vi "Photometer calibration.vi"(11 "Photometer index":i32) -> ()   [LabVIEW 2019]
uses:
  Photometer calibration data.ctl
  toolbar icons/Export pcm.ctl
  toolbar icons/Open calibration.ctl
  toolbar icons/Save calibration.ctl
  DAQ configuration/Sensor buffer command.ctl
  Process Controller 3.0/Calibration and Function folders.ctl
panel:
  in  "Tab Control":enum32{"Analysis", "Help"}(tab)
  out "Absorbance linear fit":cluster{"Best Linear Fit":dbl[], dbl[]}[](graph)
  in  "units":string
  in  "Add Standard":bool
  in  "Clear Standards":bool
  out "Voltage":sgl[unit] format="%.3f"
  out "Concentration":dbl format="%_3f"
  out "XY Graph":cluster{dbl[], dbl[]}[](graph)
  out "A":dbl format="%_3f"
  in  "data averaging (s)":sgl=5.0 format="%.1f"
  in  "Standards":cluster{"Concentration":dbl, "Voltage":dbl}[](array[cluster])=[{"Concentration"=2.0, "Voltage"=2.35551381111145}, {"Concentration"=5.0, "Voltage"=1.50419282913208}, {"Concentration"=10.0, "Voltage"=0.7342819571495056}, {"Concentration"=20.0, "Voltage"=0.23017707467079163}, {"Concentration"=50.0, "Voltage"=0.09496632218360901}] caption="Concentration                        Voltage"
  out "Dark Voltage":dbl=0.09145960211753845
  out "Blank Voltage":dbl=3.127514600753784
  in  "Read\nStandard":bool[](array[boolean])
  in  "Read Dark":bool
  in  "Read Blank":bool
  in  "OK Button":bool
  in  "Cancel":bool
  out "slope":dbl
  out "intercept":dbl
  out "R-square":dbl
  in  "export":T1
  in  "Open calibration":T2
  in  "Save calibration":T3
  out "Photometer data in":T4
  out "Quit":bool
  # "Dark voltage is obtained by turning off the LED light or by completely blocking the sensor. Use an opaque object (not your finger).\nBlank is the same as a standard with zero concentration of the constituent that is being measured.\n\nYou can add or delete standards by right clicking and selecting Insert Element Before or Delete Element."
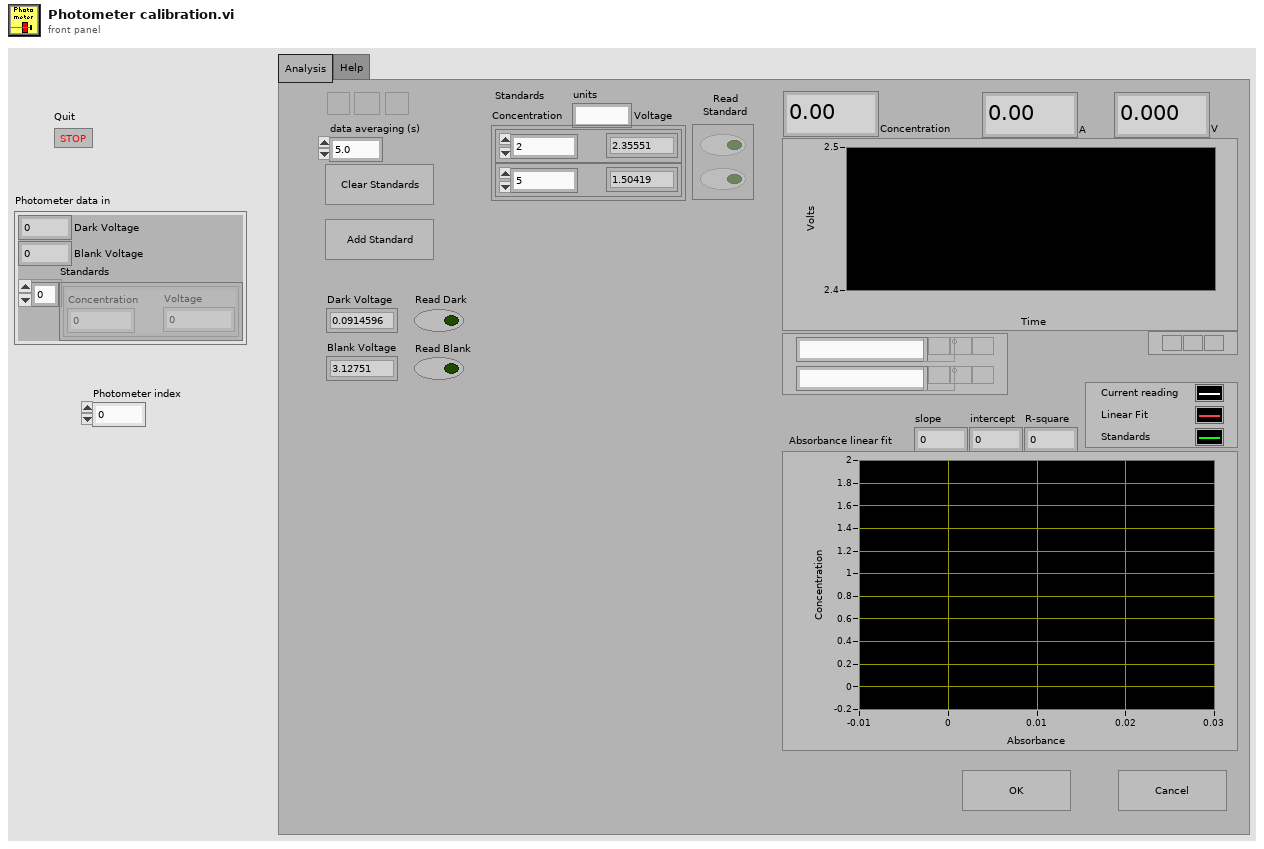
[diagram p1: front panel]
types:
  T1 = typedef "Export pcm.ctl" = bool
  T2 = typedef "Open calibration.ctl" = bool
  T3 = typedef "Save calibration.ctl" = bool
  T4 = typedef "Photometer calibration data.ctl" = cluster{"Dark Voltage":dbl, "Blank Voltage":dbl, "Standards":cluster{"Concentration":dbl, "Voltage":dbl}[]}
  T5 = typedef "Sensor buffer command.ctl" = enum16{"read average", "read recent", "read all", "write", "set buffer size", "Read channel config", "Write channel config", "clear"}
  T6 = typedef "Calibration and Function folders.ctl" = enum16{"Sensors", "Functions", "Config File", "PublicAppFolder", "New ini File", "Set Config File", "Delete ini File"}
  T7 = typedef "Channel config.ctl" = cluster{"Channel Indices":T8[], "AI Max voltage":dbl[], "Calibration matrix":T9}
  T8 = typedef "channel identifier.ctl" = u16
  T9 = typedef "calib array.ctl" = T10[]
  T10 = typedef "conversion.ctl" = cluster{"conversion matrix":sgl[][], "units":string, "name":string, "scale type":T11, "offset (volts)":dbl, "second channel":i8, "correspondence table":T12, "offset (physical units)":dbl, "pH scale":T13, "D.O.":T14, "Photometer data":T4}
  T11 = typedef "scale type.ctl" = enum16{"Volts", "Polynomial", "Correspondence Table", "pH", "Dissolved Oxygen", "Quadratic", "Photometer"}
  T12 = typedef "correspondence table.ctl" = cluster{"physical units":dbl, "volts":dbl}[]
  T13 = typedef "pH scale.ctl" = cluster{"Buffers":cluster{"Buffer":dbl, "Calibrated":bool, "V/T":dbl}[], "Temperature":dbl}
  T14 = typedef "DO scale.ctl" = cluster{"Temperature":dbl, "K":dbl, "barometric pressure":dbl}
  T15 = typedef "Sensor data.ctl" = cluster{" Sensor array":T16[], "Time":dbl}
  T16 = typedef "sensor cluster.ctl" = cluster{"voltage":sgl, "scaled":sgl, "units":string, "Out of Range":bool}
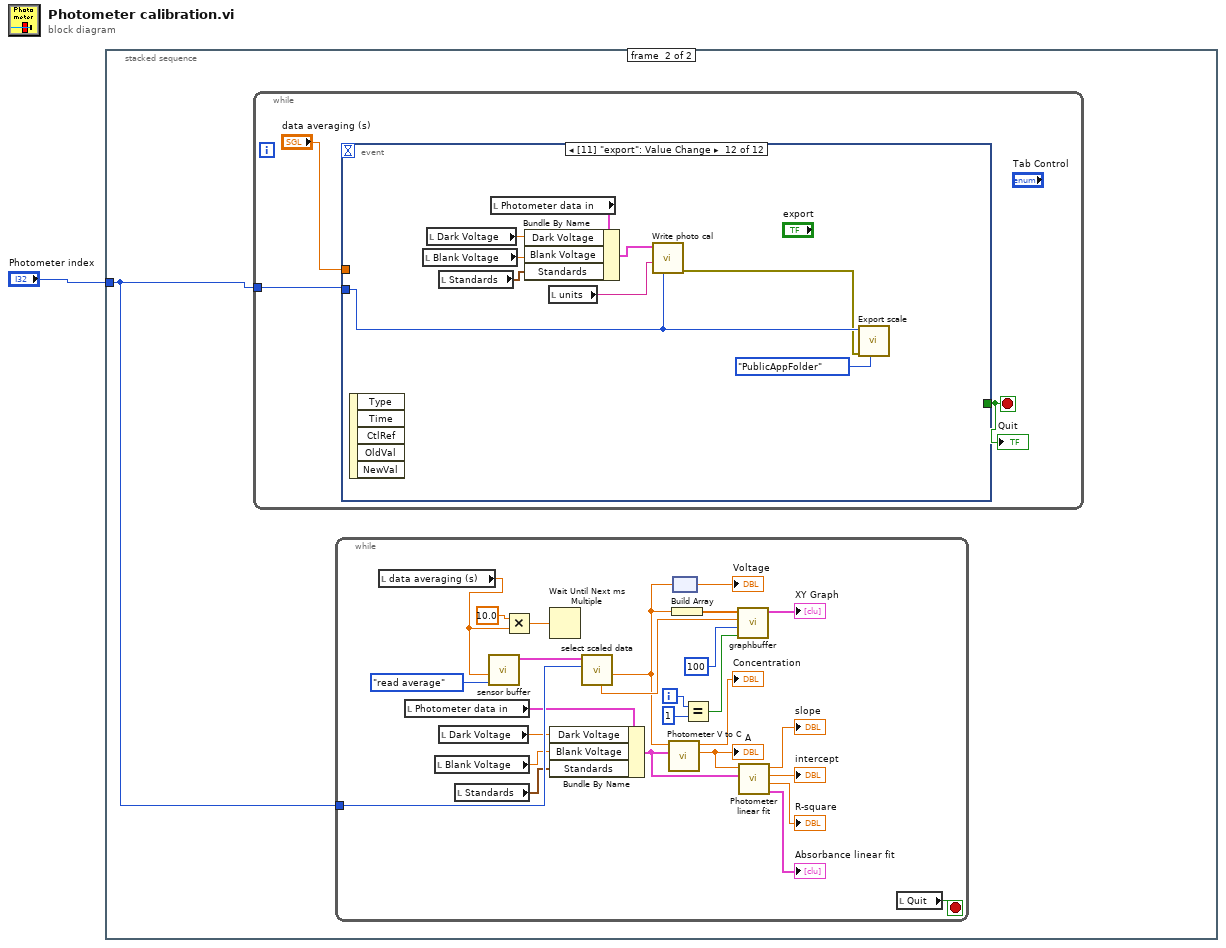
[diagram p0: block diagram]
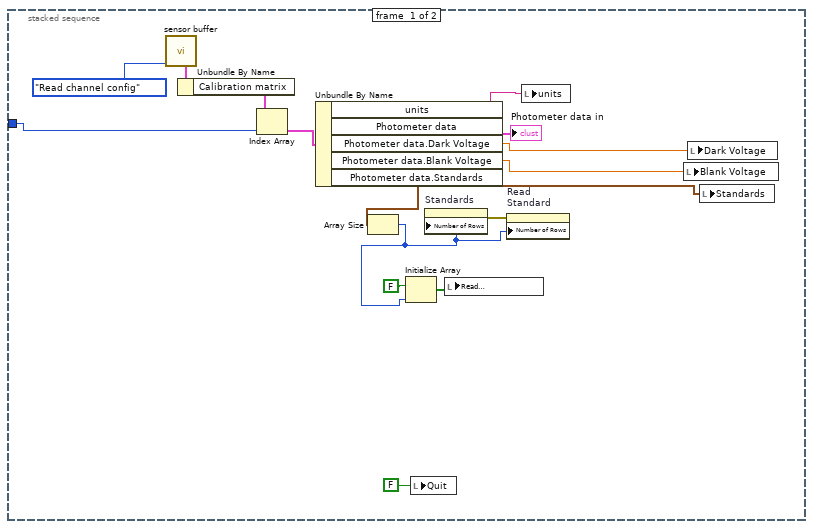
[diagram p2: hidden frame]
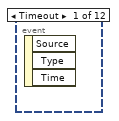
[diagram p3: hidden frame]
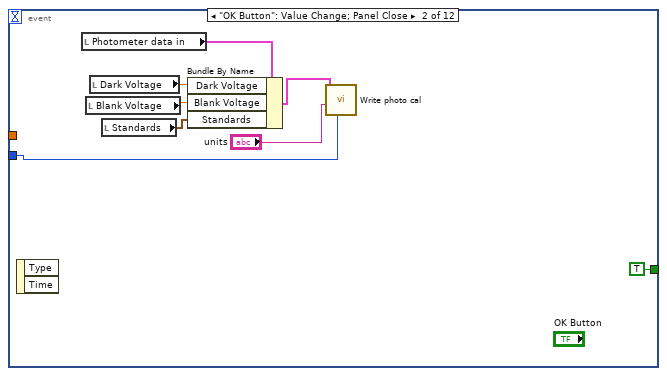
[diagram p4: hidden frame]
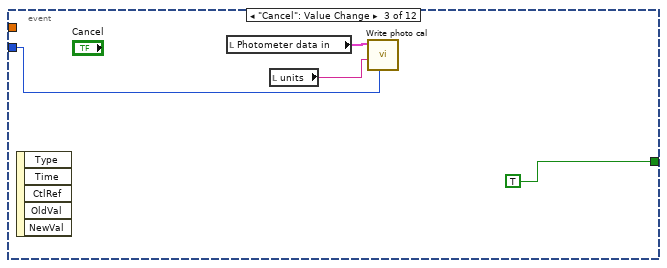
[diagram p5: hidden frame]
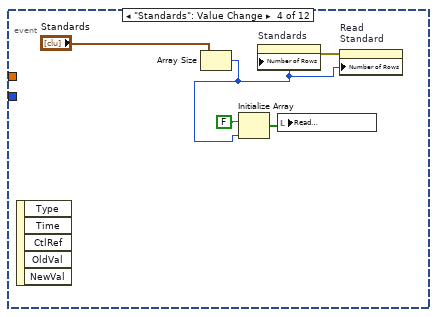
[diagram p6: hidden frame]
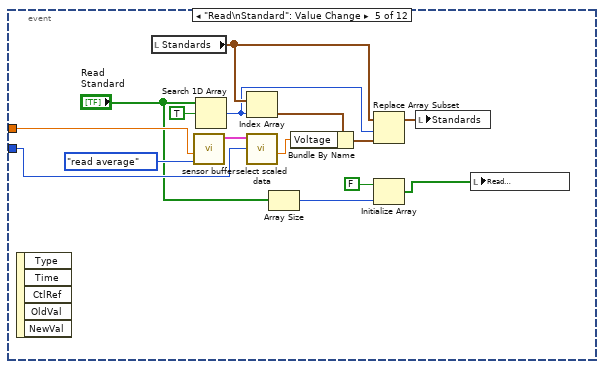
[diagram p7: hidden frame]
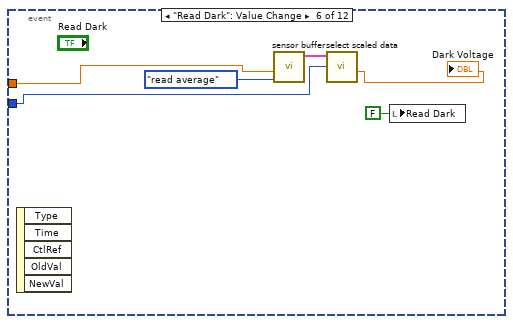
[diagram p8: hidden frame]
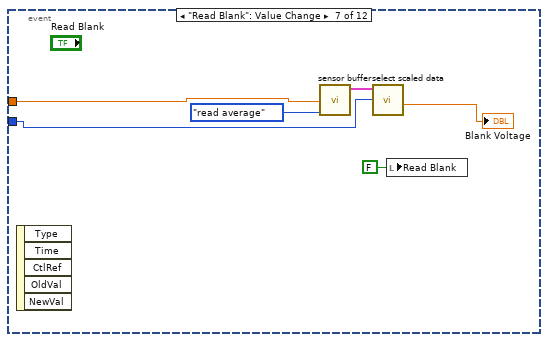
[diagram p9: hidden frame]
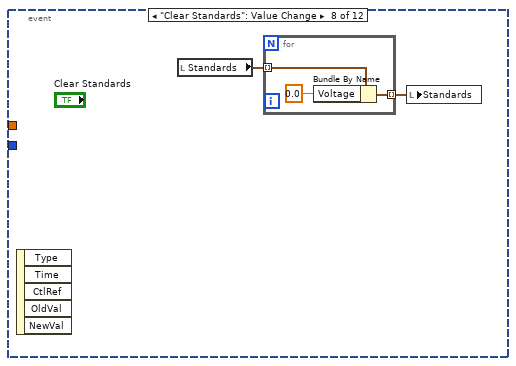
[diagram p10: hidden frame]
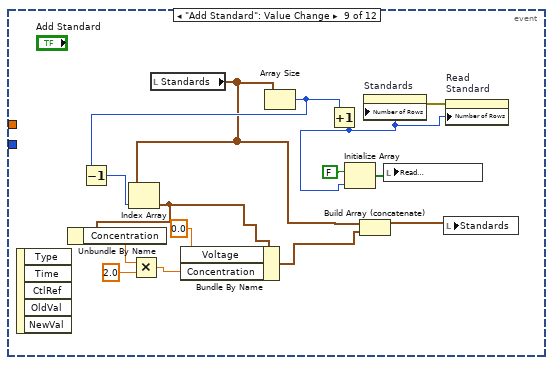
[diagram p11: hidden frame]
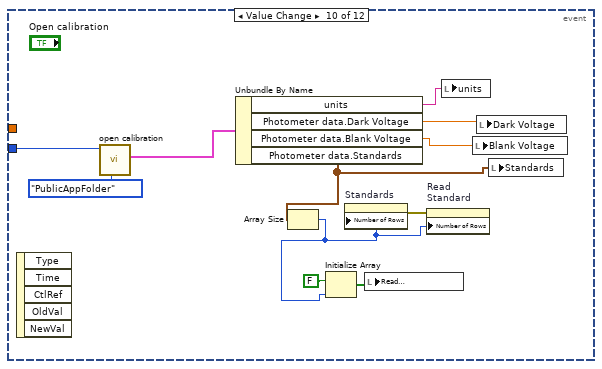
[diagram p12: hidden frame]
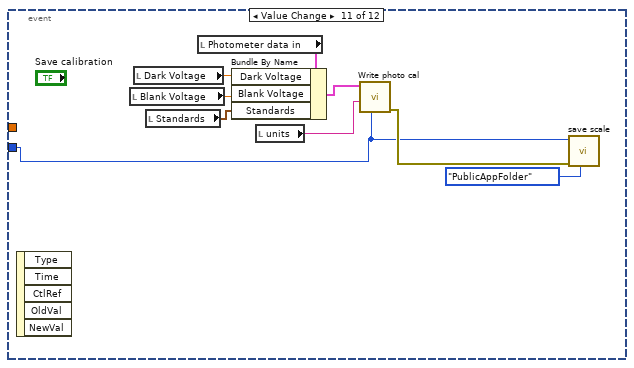
[diagram p13: hidden frame]
diagram:
  n1 = stacked-sequence {
    tunnel: "Photometer index" -> [w12 w17]
    frame #0 {
      n2 = call "sensor buffer.vi"("command"=Sensor_buffer_command."Read channel config") -> ("Channel Config out"=w14:T7)  [unwired: 6 in, 4 out]
      n3 = Unbundle By Name(w14) -> ("Calibration matrix"=w13:T9)
      n4 = Index Array(array=w13, index=w12) -> (element=w11:T10)
      n5 = Unbundle By Name(w11) -> ("units"=w5:string, "Photometer data"=→"Photometer data in":T4, "Photometer data.Dark Voltage"=w3:dbl, "Photometer data.Blank Voltage"=w2:dbl, "Photometer data.Standards"=w4:cluster{"Concentration":dbl, "Voltage":dbl}[])
      n6 = Array Size(array=w4) -> (size(s)=w6:i32)
      n7 = Initialize Array(FALSE, w6) -> (w8:bool[])
      n8 = local write "Quit"(FALSE ("Quit")) -> ()
      n9 = property on="Standards" class="Arr (strict)"("Number of Rows"=w6) -> (error out=w7:errorcluster)  [unwired: 2 in, 1 out]
      n10 = local write "Read\nStandard"(w8) -> ()
      n11 = property on="Read\nStandard" class="Arr (strict)"(error in=w7, "Number of Rows"=w6) -> ()  [unwired: 1 in, 2 out]
      n12 = local write "units"(w5) -> ()
      n13 = local write "Blank Voltage"(w2) -> ()
      n14 = local write "Dark Voltage"(w3) -> ()
      n15 = local write "Standards"(w4) -> ()
    }
    frame #1 {
      n16 = while {
        tunnel: w17 -> [w46]
        stop <- w47 stop-if-true
        n17 = event shown="[11] \"export\": Value Change" {
          selector: _ -> [_ _ _ _ _ _ _ _ _ _ _ _]
          dyn-events: _ -> [_ _ _ _ _ _ _ _ _ _ _ _]
          timeout: _ -> [_ _ _ _ _ _ _ _ _ _ _ _]
          tunnel: [_ TRUE ("OK Button") TRUE ("OK Button") _ _ _ _ _ _ _ _ _] -> w47
          tunnel: w46 -> [_ w54 w56 _ w77 w83 w88 _ _ w116 w127 w132]
          tunnel: "data averaging (s)" -> [_ _ _ _ w69 w81 w87 _ _ _ _ _]
          event Timeout {
            n18 = event-data() -> ()  [unwired: 1 in, 3 out]
          }
          event "OK Button": Value Change; Panel Close {
            n19 = event-data() -> ()  [unwired: 1 in, 2 out]
            n20 = local read "Photometer data in"() -> (w53:T4)
            n21 = local read "Blank Voltage"() -> (w49:dbl)
            n22 = local read "Dark Voltage"() -> (w50:dbl)
            n23 = local read "Standards"() -> (w48:cluster{"Concentration":dbl, "Voltage":dbl}[])
            n24 = Bundle By Name(cluster=w53, "Dark Voltage"=w50, "Blank Voltage"=w49, "Standards"=w48) -> (w51:T4)
            n25 = call "Write photo cal.vi"("Photometer index"=w54, "units"="units", "Photometer data in"=w51) -> ()  [unwired: 8 in, 1 out]
          }
          event "Cancel": Value Change {
            n26 = event-data() -> ()  [unwired: 1 in, 5 out]
            n27 = local read "Photometer data in"() -> (w58:T4)
            n28 = local read "units"() -> (w57:string)
            n29 = call "Write photo cal.vi"("Photometer index"=w56, "units"=w57, "Photometer data in"=w58) -> ()  [unwired: 8 in, 1 out]
          }
          event "Standards": Value Change {
            n30 = event-data() -> ()  [unwired: 1 in, 5 out]
            n31 = Array Size(array="Standards") -> (size(s)=w60:i32)
            n32 = Initialize Array(FALSE, w60) -> (w62:bool[])
            n33 = property on="Standards" class="Arr (strict)"("Number of Rows"=w60) -> (error out=w61:errorcluster)  [unwired: 2 in, 1 out]
            n34 = local write "Read\nStandard"(w62) -> ()
            n35 = property on="Read\nStandard" class="Arr (strict)"(error in=w61, "Number of Rows"=w60) -> ()  [unwired: 1 in, 2 out]
          }
          event "Read\nStandard": Value Change {
            n36 = event-data() -> ()  [unwired: 1 in, 5 out]
            n37 = local read "Standards"() -> (w74:cluster{"Concentration":dbl, "Voltage":dbl}[])
            n38 = call "sensor buffer.vi"("command"=Sensor_buffer_command."read average", "smooth interval (s)"=w69) -> ("Calibrated data"=w78:T15)  [unwired: 5 in, 4 out]
            n39 = Search 1D Array(1D array="Read\nStandard", element=TRUE) -> (index of element=w73:i32)  [unwired: 1 in]
            n40 = Index Array(array=w74, index=w73) -> (element=w72:cluster{"Concentration":dbl, "Voltage":dbl})
            n41 = call "select scaled data.vi"("Sensor index"=w77, "Sensor Data"=w78) -> ("voltage"=w71:sgl)  [unwired: 4 in, 5 out]
            n42 = Array Size(array="Read\nStandard") -> (size(s)=w67:i32)
            n43 = Bundle By Name(cluster=w72, "Voltage"=w71) -> (w70:cluster{"Concentration":dbl, "Voltage":dbl})
            n44 = Replace Array Subset(array=w74, new element=w70, index=w73) -> (w75:cluster{"Concentration":dbl, "Voltage":dbl}[])
            n45 = Initialize Array(FALSE ("element"), w67) -> (w66:bool[])
            n46 = local write "Standards"(w75) -> ()
            n47 = local write "Read\nStandard"(w66) -> ()
          }
          event "Read Dark": Value Change {
            n48 = event-data() -> ()  [unwired: 1 in, 5 out]
            n49 = call "sensor buffer.vi"("command"=Sensor_buffer_command."read average", "smooth interval (s)"=w81) -> ("Calibrated data"=w85:T15)  [unwired: 5 in, 4 out]
            n50 = call "select scaled data.vi"("Sensor index"=w83, "Sensor Data"=w85) -> ("voltage"=→"Dark Voltage":sgl)  [unwired: 4 in, 5 out]
            n51 = local write "Read Dark"(FALSE ("Read Dark")) -> ()
          }
          event "Read Blank": Value Change {
            n52 = event-data() -> ()  [unwired: 1 in, 5 out]
            n53 = call "sensor buffer.vi"("command"=Sensor_buffer_command."read average", "smooth interval (s)"=w87) -> ("Calibrated data"=w91:T15)  [unwired: 5 in, 4 out]
            n54 = call "select scaled data.vi"("Sensor index"=w88, "Sensor Data"=w91) -> ("voltage"=→"Blank Voltage":sgl)  [unwired: 4 in, 5 out]
            n55 = local write "Read Blank"(FALSE ("Read Blank")) -> ()
          }
          event "Clear Standards": Value Change {
            n56 = event-data() -> ()  [unwired: 1 in, 5 out]
            n57 = local read "Standards"() -> (w93:cluster{"Concentration":dbl, "Voltage":dbl}[])
            n58 = for {
              tunnel: w93 -> [w96] mode=indexing
              tunnel: [w94] -> w92 mode=indexing
              n59 = Bundle By Name(cluster=w96, "Voltage"=0.0) -> (w94:cluster{"Concentration":dbl, "Voltage":dbl})
            }
            n60 = local write "Standards"(w92) -> ()
          }
          event "Add Standard": Value Change {
            n61 = event-data() -> ()  [unwired: 1 in, 5 out]
            n62 = local read "Standards"() -> (w100:cluster{"Concentration":dbl, "Voltage":dbl}[])
            n63 = Array Size(array=w100) -> (size(s)=w102:i32)
            n64 = Decrement(x=w102) -> (x-1=w97:i32)
            n65 = Index Array(array=w100, index=w97) -> (element=w106:cluster{"Concentration":dbl, "Voltage":dbl})
            n66 = Unbundle By Name(w106) -> ("Concentration"=w105:dbl)
            n67 = Multiply(x=w105, y=2.0) -> (x*y=w103:dbl)
            n68 = Bundle By Name(cluster=w106, "Voltage"=0.0, "Concentration"=w103) -> (w98:cluster{"Concentration":dbl, "Voltage":dbl})
            n69 = Increment(x=w102) -> (x+1=w101:i32)
            n70 = Initialize Array(FALSE, w101) -> (w109:bool[])
            n71 = Build Array (concatenate)(w100, w98) -> (w99:cluster{"Concentration":dbl, "Voltage":dbl}[])
            n72 = property on="Standards" class="Arr (strict)"("Number of Rows"=w101) -> (error out=w108:errorcluster)  [unwired: 2 in, 1 out]
            n73 = local write "Read\nStandard"(w109) -> ()
            n74 = local write "Standards"(w99) -> ()
            n75 = property on="Read\nStandard" class="Arr (strict)"(error in=w108, "Number of Rows"=w101) -> ()  [unwired: 1 in, 2 out]
          }
          event Value Change {
            n76 = event-data() -> ()  [unwired: 1 in, 5 out]
            n77 = call "open calibration.vi"("Folder"=Calibration_and_Function_folders."PublicAppFolder", "Index"=w116) -> ("conversion out"=w115:T10)  [unwired: 7 in, 2 out]
            n78 = Unbundle By Name(w115) -> ("units"=w114:string, "Photometer data.Dark Voltage"=w113:dbl, "Photometer data.Blank Voltage"=w112:dbl, "Photometer data.Standards"=w111:cluster{"Concentration":dbl, "Voltage":dbl}[])
            n79 = Array Size(array=w111) -> (size(s)=w117:i32)
            n80 = Initialize Array(FALSE, w117) -> (w119:bool[])
            n81 = property on="Standards" class="Arr (strict)"("Number of Rows"=w117) -> (error out=w118:errorcluster)  [unwired: 2 in, 1 out]
            n82 = local write "Read\nStandard"(w119) -> ()
            n83 = property on="Read\nStandard" class="Arr (strict)"(error in=w118, "Number of Rows"=w117) -> ()  [unwired: 1 in, 2 out]
            n84 = local write "units"(w114) -> ()
            n85 = local write "Blank Voltage"(w112) -> ()
            n86 = local write "Dark Voltage"(w113) -> ()
            n87 = local write "Standards"(w111) -> ()
          }
          event Value Change {
            n88 = event-data() -> ()  [unwired: 1 in, 5 out]
            n89 = local read "Blank Voltage"() -> (w123:dbl)
            n90 = local read "Dark Voltage"() -> (w124:dbl)
            n91 = local read "Standards"() -> (w129:cluster{"Concentration":dbl, "Voltage":dbl}[])
            n92 = local read "Photometer data in"() -> (w125:T4)
            n93 = Bundle By Name(cluster=w125, "Dark Voltage"=w124, "Blank Voltage"=w123, "Standards"=w129) -> (w126:T4)
            n94 = local read "units"() -> (w122:string)
            n95 = call "Write photo cal.vi"("Photometer index"=w127, "units"=w122, "Photometer data in"=w126) -> ("error out"=w128:errorcluster)  [unwired: 8 in]
            n96 = call "save scale.vi"("Folder"=Calibration_and_Function_folders."PublicAppFolder", "error in (no error)"=w128, "Index"=w127) -> ()  [unwired: 7 in, 1 out]
          }
          event Value Change {
            n97 = event-data() -> ()  [unwired: 1 in, 5 out]
            n98 = local read "Blank Voltage"() -> (w134:dbl)
            n99 = local read "Dark Voltage"() -> (w135:dbl)
            n100 = local read "Standards"() -> (w138:cluster{"Concentration":dbl, "Voltage":dbl}[])
            n101 = local read "Photometer data in"() -> (w136:T4)
            n102 = Bundle By Name(cluster=w136, "Dark Voltage"=w135, "Blank Voltage"=w134, "Standards"=w138) -> (w137:T4)
            n103 = local read "units"() -> (w133:string)
            n104 = call "Write photo cal.vi"("Photometer index"=w132, "units"=w133, "Photometer data in"=w137) -> ("error out"=w131:errorcluster)  [unwired: 8 in]
            n105 = call "Export scale.vi"("Folder"=Calibration_and_Function_folders."PublicAppFolder", "error in (no error)"=w131, "Index"=w132) -> ()  [unwired: 7 in, 1 out]
          }
        }
        "Quit" <- w47
      }
      n106 = while {
        tunnel: w17 -> [w36]
        i -> [w35]
        stop <- w44 stop-if-true
        n107 = local read "data averaging (s)"() -> (w18:sgl)
        n108 = local read "Photometer data in"() -> (w26:T4)
        n109 = local read "Blank Voltage"() -> (w27:dbl)
        n110 = local read "Dark Voltage"() -> (w28:dbl)
        n111 = local read "Standards"() -> (w29:cluster{"Concentration":dbl, "Voltage":dbl}[])
        n112 = call "sensor buffer.vi"("command"=Sensor_buffer_command."read average", "smooth interval (s)"=w18) -> ("Calibrated data"=w32:T15)  [unwired: 5 in, 4 out]
        n113 = Multiply(x=10.0 ("y"), y=w18) -> (x*y=w43:dbl)
        n114 = Wait Until Next ms Multiple(millisecond multiple=w43) -> ()  [unwired: 1 out]
        n115 = Bundle By Name(cluster=w26, "Dark Voltage"=w28, "Blank Voltage"=w27, "Standards"=w29) -> (w24:T4)
        n116 = call "select scaled data.vi"("Sensor index"=w36, "Sensor Data"=w32) -> ("voltage"=w30:sgl, "Time"=w41:dbl)  [unwired: 4 in, 4 out]
        n117 = call "Photometer V to C.vi"("Photometer data in"=w24, "Volts"=w30) -> ("Absorbance"=w23:dbl, "Concentration"=→"Concentration":dbl)  [unwired: 8 in]
        "A" <- w23
        n118 = Build Array(w30) -> (w31:sgl[])
        n119 = node(w30) -> (→"Voltage":sgl[unit])
        n120 = Equal?(x=w35, y=1) -> (x = y?=w39:bool)
        n121 = call "graphbuffer.vi"("Reset"=w39, "history length"=u16 100, "Time"=w41, "data"=w31) -> ("Multiplot graph data"=→"XY Graph":cluster{dbl[], dbl[]}[])  [unwired: 5 in, 2 out]
        n122 = call "Photometer linear fit.vi"("Photometer data in"=w24, "Absorbance"=w23) -> ("XY Graph"=→"Absorbance linear fit":cluster{"Best Linear Fit":dbl[], dbl[]}[], "R-square"=→"R-square":dbl, "intercept"=→"intercept":dbl, "slope"=→"slope":dbl)  [unwired: 6 in]
        n123 = local read "Quit"() -> (w44:bool)
      }
    }
  }
